vi "Find Workspace.vi"(8 "Error In":errorcluster, 9 "Assembly Type":string, 10 "Control In":T2={"I-O.lvclass"=refnum, "Gantry"=refnum, "Dispenser"="COM1"}, 11 "Carrier Tray in":refnum<class "Assembly Tray.lvclass">) -> (0 "Error Out":errorcluster, 1 "Workspace":T1, 2 "Control Out":T2={"I-O.lvclass"=refnum, "Gantry"=refnum, "Dispenser"="COM1"}, 3 "Carrier Tray Out":refnum<class "Assembly Tray.lvclass">)   [LabVIEW 2021, in "Assembly Tray.lvclass"]
uses:
  Assembly Tray.lvclass
  C:/Users/HEP/Documents/GitHub/Gantry/UCSB-Gantry-HEP-main/Classes/Workspace/Fixture.lvclass
  Controller/Controllers.ctl
  Controller/I-O/I-O.lvclass
  C:/Program Files (x86)/Aerotech/A3200/LabVIEW/2010/Bin/Aerotech.A3200.dll
  Program Files (x86)/Aerotech/A3200/LabVIEW/2010/Bin/Aerotech.A3200.dll
  Workspace.ctl
  Fixture.lvclass/Fixture.ctl
  Assembly Tray.lvclass/Assembly Tray.ctl
  Read Fixture ID.vi
  Read Position.vi
  Fixture.lvclass
  Controller/Controller.lvclass
panel:
  out "XYZTheta Centers":dbl[][](array[numeric])
  in  "output cluster 2":T1
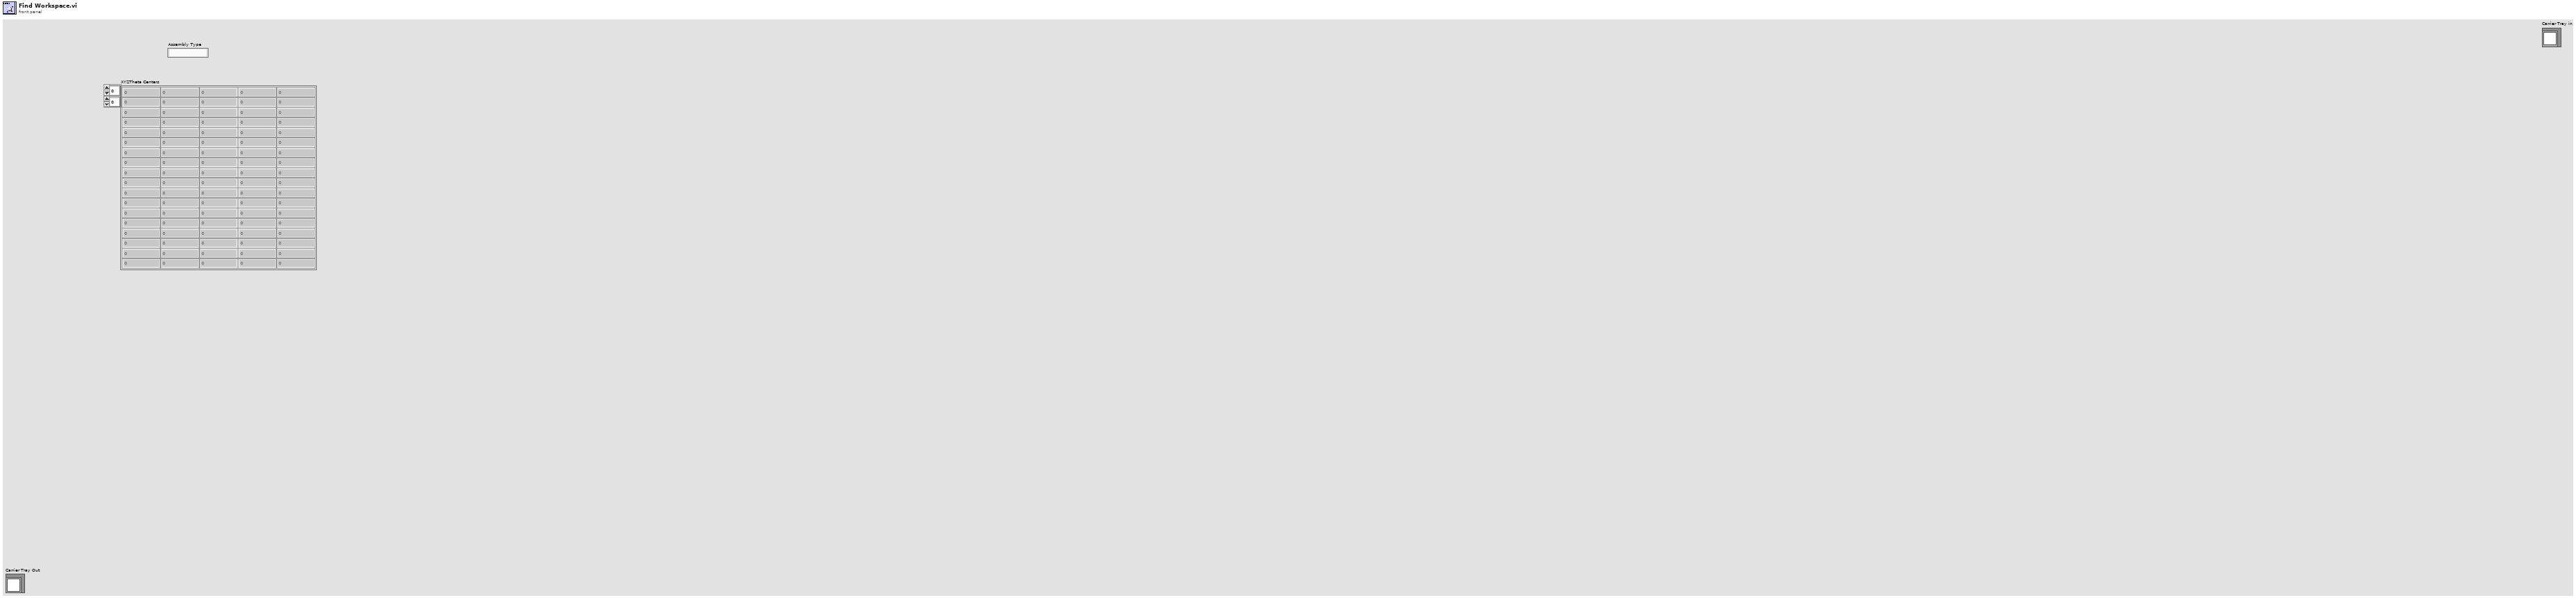
[diagram p1: front panel]
types:
  T1 = typedef "Fixture.lvclass/Workspace.ctl" = cluster{"XYZTheta":dbl[], "Workspace Valve":i32, "Workspace Sensor":i32}
  T2 = typedef "Controller.lvclass/Controllers.ctl" = cluster{"I-O.lvclass":refnum<class "I-O.lvclass">, "Gantry":refnum<k24>, "Dispenser":refnum<visa-resource-name>}
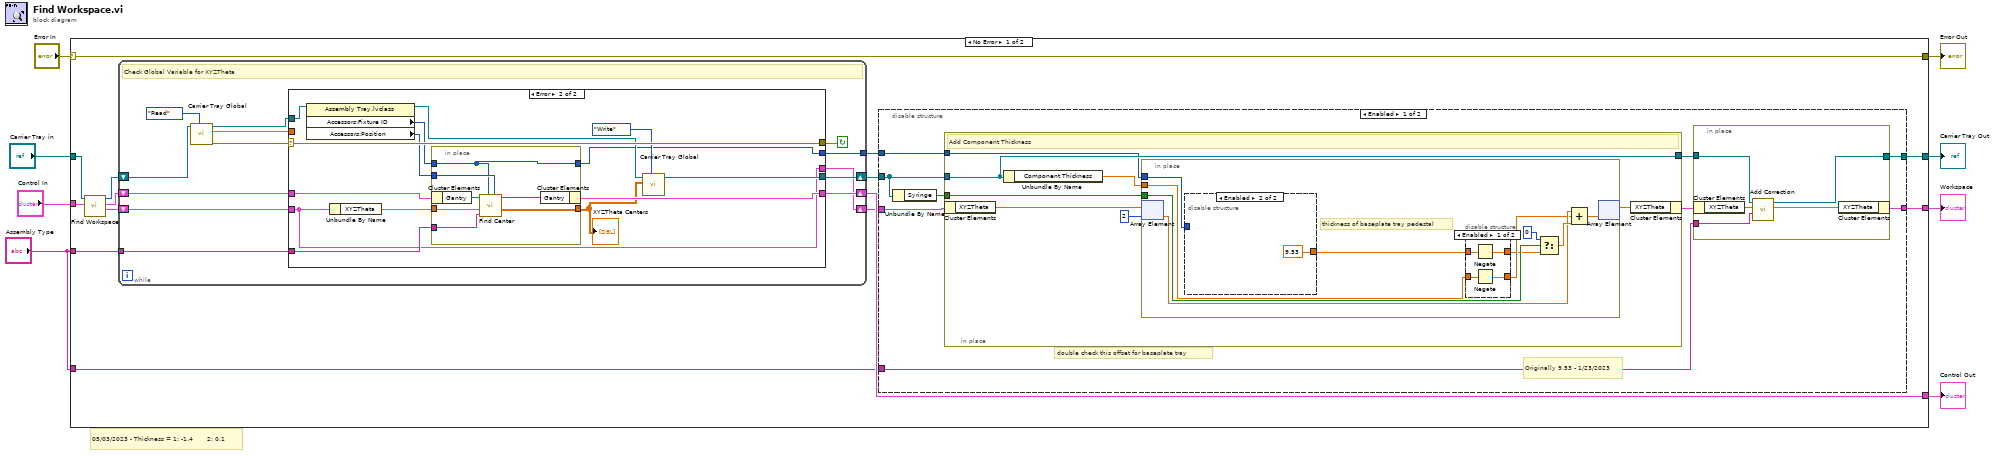
[diagram p0: block diagram]
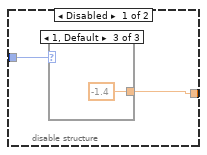
[diagram p2: hidden frame]
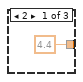
[diagram p3: hidden frame]
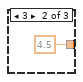
[diagram p4: hidden frame]
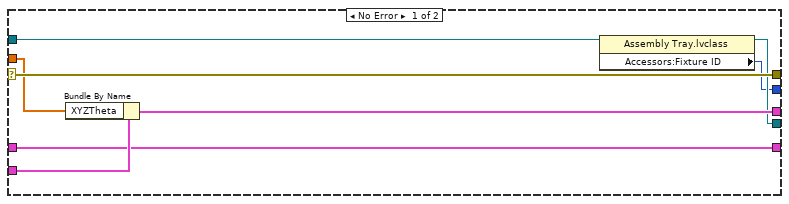
[diagram p7: hidden frame]
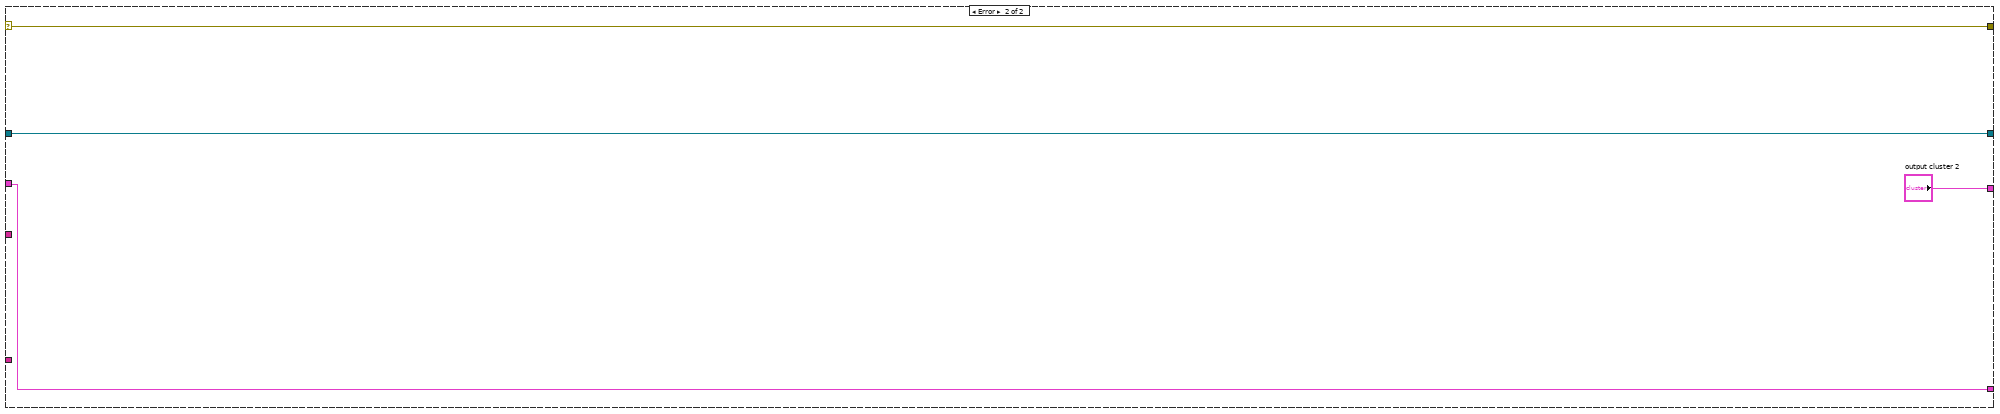
[diagram p8: hidden frame]
diagram:
  # "05/03/2023 - Thickness = 1: -1.4       2: 0.1"
  n1 = case shown="No Error" "Error In" {
    selector: "Error In" -> [w22 w112]
    tunnel: [w22 w112] -> w7
    tunnel: "Control In" -> [w21 w113]
    tunnel: [w17 w113] -> w5
    tunnel: "Carrier Tray in" -> [w20 w110]
    tunnel: [w18 "output cluster 2"] -> w3
    tunnel: [w19 w110] -> w2
    tunnel: "Assembly Type" -> [w11 _]
    tunnel: "Assembly Type" -> [w9 _]
    frame No Error {
      n2 = call-parent "Find Workspace.vi"("Control In"=w21, "Workspace In"=w20) -> (1:"Workspace Out"=w16:T1, "Control Out"=w15:T2, 3:"Workspace Out"=w12:refnum<class "Assembly Tray.lvclass">)  [unwired: 6 in, 1 out]
      n3 = while {
        shift-right: [w73] -> w14
        shift-left: w12 -> [w71]
        shift-right: [w75] -> w17
        shift-left: w15 -> [w76]
        shift-right: [w72] -> w13
        shift-left: w16 -> [w77]
        tunnel: w11 -> [w69]
        tunnel: [w68] -> w10
        stop <- w79 continue-if-true
        # "Check Global Variable for XYZTheta"
        n4 = call "Carrier Tray Global.vi"("Action"=enum16{"Initialize", "Read", "Write"}."Read", "Carrier Tray.lvclass"=w71) -> ("error out"=w70:errorcluster, "XYZTheta out"=w78:dbl[], "Carrier Tray.lvclass 2"=w74:refnum<class "Assembly Tray.lvclass">)  [unwired: 7 in]
        n5 = case shown="Error" w70 {
          selector: w70 -> [w88 w102]
          tunnel: [w88 w102] -> w79
          tunnel: w78 -> [w87 _]
          tunnel: [w86 w89] -> w72
          tunnel: w77 -> [w85 w89]
          tunnel: w76 -> [w84 w96]
          tunnel: [w84 w95] -> w75
          tunnel: w74 -> [w83 w99]
          tunnel: [w82 w101] -> w73
          tunnel: w69 -> [_ w92]
          tunnel: [w81 w90] -> w68
          frame No Error {
            n6 = Bundle By Name(cluster=w85, "XYZTheta"=w87) -> (w86:T1)
            n7 = property class="Assembly Tray.lvclass"(reference=w83) -> (reference out=w82:refnum<class "Assembly Tray.lvclass">, "Accessors:Fixture ID"=w81:i32)  [unwired: 1 in, 1 out]
          }
          frame Error {
            n8 = property class="Assembly Tray.lvclass"(reference=w99) -> (reference out=w98:refnum<class "Assembly Tray.lvclass">, "Accessors:Fixture ID"=w97:i32, "Accessors:Position"=w91:i32)  [unwired: 1 in, 1 out]
            n9 = Unbundle By Name(w89) -> ("XYZTheta"=w94:dbl[])
            n10 = in-place {
              in-place-border: w97 -> [w103]
              in-place-border: w94 -> [w107]
              in-place-border: [w106] -> w93
              in-place-border: w92 -> [w105]
              in-place-border: w91 -> [w104]
              in-place-border: [w103] -> w90
              n11 = in-place-cluster #1(w96) -> ("Gantry"=w109:refnum<k24>)
              n12 = call "Find Center.vi"("Position"=w104, "Tray Number"=w103, "Assembly Type"=w105, "XYZTheta"=w107, "Gantry In"=w109) -> ("XYZTheta Centers"=w106:dbl[][], "Gantry Out"=w108:refnum<k24>)  [unwired: 5 in]
              n13 = in-place-cluster #1("Gantry"=w108) -> (w95:T2)
            }
            "XYZTheta Centers" <- w93
            n14 = call "Carrier Tray Global.vi"("Action"=enum16{"Initialize", "Read", "Write"}."Write", "XYZTheta in"=w93, "Carrier Tray.lvclass"=w98) -> ("Carrier Tray.lvclass 2"=w101:refnum<class "Assembly Tray.lvclass">)  [unwired: 6 in, 2 out]
          }
        }
      }
      n15 = disable-structure shown="Enabled" {
        disable-tunnel: [w31 w66] -> w19
        disable-tunnel: [w30 w67] -> w18
        disable-tunnel: w14 -> [w29 w66]
        disable-tunnel: w13 -> [w28 w67]
        disable-tunnel: w10 -> [w24 _]
        disable-tunnel: w9 -> [w23 _]
        frame Enabled {
          # "Originally 9.53 - 1/23/2023"
          # "double check this offset for baseplate tray"
          n16 = Unbundle By Name(w29) -> ("Syringe"=w27:bool)
          n17 = in-place {
            in-place-border: w29 -> [w41]
            in-place-border: [w41] -> w26
            in-place-border: w27 -> [w40]
            in-place-border: w24 -> [w38]
            # "Add Component Thickness"
            n18 = in-place-cluster #2(w28) -> ("XYZTheta"=w39:dbl[])
            n19 = Unbundle By Name(w41) -> ("Component Thickness"=w42:dbl)
            n20 = in-place {
              in-place-border: w42 -> [w48]
              in-place-border: w40 -> [w52]
              in-place-border: w38 -> [w44]
              # "thickness of baseplate tray pedestal"
              n21 = in-place-array #3(w39, 2) -> (w49:dbl)
              n22 = disable-structure shown="Enabled" {
                disable-tunnel: [w55 9.53] -> w46
                disable-tunnel: w44 -> [w54 _]
                frame Disabled {
                  n23 = case shown="1, Default" w54 {
                    tunnel: [4.4 4.5 -1.4] -> w55
                    frame 2 {
                    }
                    frame 3 {
                    }
                    frame 1, Default {
                    }
                  }
                }
                frame Enabled {
                }
              }
              n24 = disable-structure shown="Enabled" {
                disable-tunnel: w48 -> [w63 w65]
                disable-tunnel: [w62 w65] -> w47
                disable-tunnel: w46 -> [w61 w64]
                disable-tunnel: [w60 w64] -> w45
                frame Enabled {
                  n25 = Negate(x=w61) -> (-x=w60:dbl)
                  n26 = Negate(x=w63) -> (-x=w62:dbl)
                }
                frame Disabled {
                }
              }
              n27 = Select(t=0, s=w52, f=w45) -> (s? t:f=w50:dbl)
              n28 = Compound Arithmetic op=ADD(w49, w47, w50) -> (w53:dbl)
              n29 = in-place-array #3(w53) -> (w43:dbl[])  [unwired: 1 out]
            }
            n30 = in-place-cluster #2("XYZTheta"=w43) -> (w25:T1)
          }
          n31 = in-place {
            in-place-border: [w36] -> w31
            in-place-border: w26 -> [w35]
            in-place-border: w23 -> [w32]
            n32 = in-place-cluster #4(w25) -> ("XYZTheta"=w34:dbl[])
            n33 = call "Add Correction.vi"("Assembly Type"=w32, "XYZTheta"=w34, "Carrier Tray in"=w35) -> ("XYZTheta Out"=w33:dbl[], "Carrier Tray out"=w36:refnum<class "Assembly Tray.lvclass">)  [unwired: 6 in, 1 out]
            n34 = in-place-cluster #4("XYZTheta"=w33) -> (w30:T1)
          }
        }
        frame Disabled {
        }
      }
    }
    frame Error {
    }
  }
  "Error Out" <- w7
  "Control Out" <- w5
  "Workspace" <- w3
  "Carrier Tray Out" <- w2
